vi "CSM TCP-Router Client Console.vi"   [LabVIEW 2020]
uses:
  _TCP-Router Client Console/Client Console.vi
  _TCP-Router Client Console/TCP-Router Client Console.lvlib
types:
  T1 = enum32{"Bad", "Idle", "Run top level", "Running"}
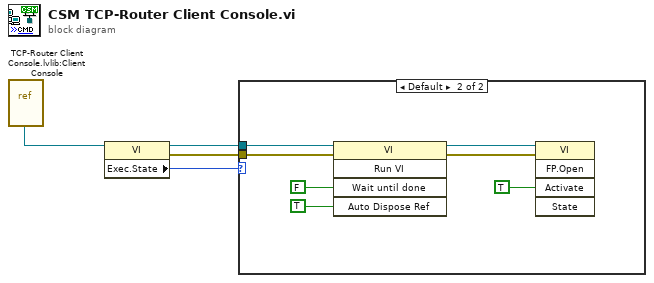
[diagram p0: block diagram]
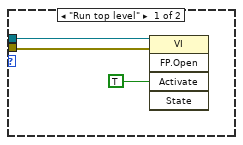
[diagram p2: hidden frame]
diagram:
  n1 = vi-ref "TCP-Router Client Console.lvlib:Client Console.vi"() -> (w4:refnum<vi>)
  n2 = property class="VI"(reference=w4) -> (reference out=w2:refnum<vi>, error out=w1:errorcluster, "Exec.State"=w3:T1)  [unwired: 1 in]
  n3 = case shown="Default" w3 {
    tunnel: w2 -> [w6 w14]
    tunnel: w1 -> [w7 w13]
    frame "Run top level" {
      n4 = invoke class="VI" method="FP.Open"(reference=w6, error in=w7, "Activate"=TRUE ("Activate?")) -> ()  [unwired: 2 in, 5 out]
    }
    frame Default {
      n5 = invoke class="VI" method="Run VI"(reference=w14, error in=w13, "Wait until done"=FALSE ("Wait Until Done"), "Auto Dispose Ref"=TRUE ("Auto Dispose Reference")) -> (reference out=w10:refnum<vi>, error out=w9:errorcluster)  [unwired: 1 in, 3 out]
      n6 = invoke class="VI" method="FP.Open"(reference=w10, error in=w9, "Activate"=TRUE ("Activate?")) -> ()  [unwired: 2 in, 5 out]
    }
  }
